vi "副屏设置.vi"() -> ()   [LabVIEW 2016, in "副屏.lvlib"]
uses:
  <vilib>/Utility/config.llb/NI_LVConfig.lvlib
panel:
  in  "ORP":bool caption="氨氮禁用"
  in  "启用副屏":bool=TRUE caption="氨氮禁用"
  in  "关闭":bool
  in  "底部状态栏显示信息":string="一体化微型水质监测系统"
  in  "流速":bool caption="氨氮禁用"
  in  "瞬时流量":bool caption="氨氮禁用"
  in  "湿度":bool=TRUE caption="氨氮禁用"
  in  "水位":bool caption="氨氮禁用"
  in  "室温":bool=TRUE caption="氨氮禁用"
  in  "CODCr":bool caption="氨氮禁用"
  in  "CODMn":bool caption="氨氮禁用"
  in  "总氮":bool caption="氨氮禁用"
  in  "总磷":bool caption="氨氮禁用"
  in  "氨氮":bool caption="氨氮禁用"
  in  "Turb":bool caption="氨氮禁用"
  in  "Cond":bool caption="氨氮禁用"
  in  "DO":bool caption="氨氮禁用"
  in  "pH":bool caption="氨氮禁用"
  in  "水温":bool caption="氨氮禁用"
  # "副屏显示信息设置"
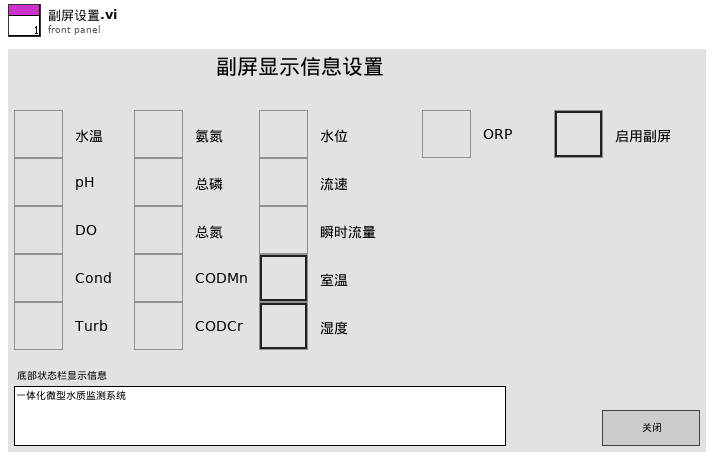
[diagram p1: front panel]
types:
  T1 = typedef "NI_LVConfig.lvlib/Config Data RefNum.ctl" = refnum<k1>
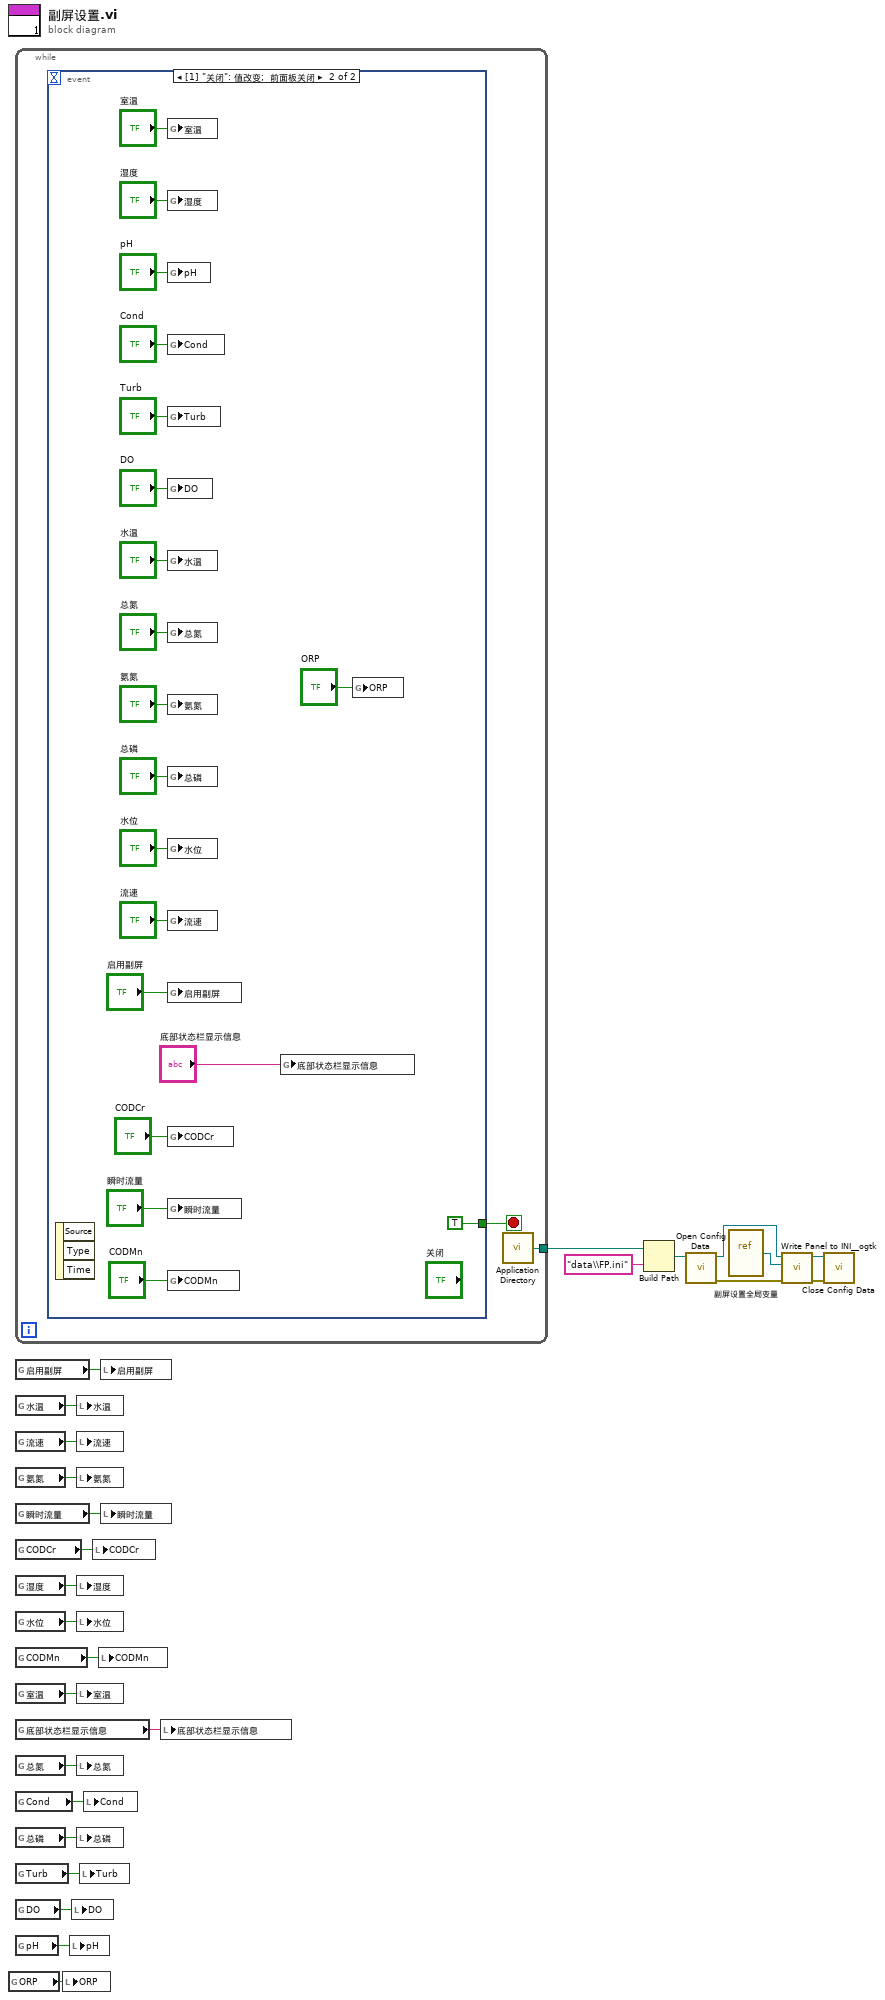
[diagram p0: block diagram]
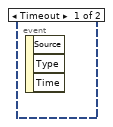
[diagram p2: hidden frame]
diagram:
  n1 = global read "副屏设置全局变量.vi" "ORP"() -> (w1:bool)
  n2 = while {
    tunnel: [w27] -> w3
    stop <- w28 stop-if-true
    n3 = event shown="[1] \"关闭\": 值改变;  前面板关闭" {
      selector: _ -> [_ _]
      dyn-events: _ -> [_ _]
      timeout: _ -> [_ _]
      tunnel: [_ TRUE] -> w28
      event Timeout {
        n4 = event-data() -> ()  [unwired: 1 in, 3 out]
      }
      event "关闭": Value Change; Panel Close {
        n5 = event-data() -> ()  [unwired: 1 in, 3 out]
        n6 = global write "副屏设置全局变量.vi" "室温"("室温") -> ()
        n7 = global write "副屏设置全局变量.vi" "湿度"("湿度") -> ()
        n8 = global write "副屏设置全局变量.vi" "pH"("pH") -> ()
        n9 = global write "副屏设置全局变量.vi" "Cond"("Cond") -> ()
        n10 = global write "副屏设置全局变量.vi" "Turb"("Turb") -> ()
        n11 = global write "副屏设置全局变量.vi" "DO"("DO") -> ()
        n12 = global write "副屏设置全局变量.vi" "水温"("水温") -> ()
        n13 = global write "副屏设置全局变量.vi" "总氮"("总氮") -> ()
        n14 = global write "副屏设置全局变量.vi" "氨氮"("氨氮") -> ()
        n15 = global write "副屏设置全局变量.vi" "总磷"("总磷") -> ()
        n16 = global write "副屏设置全局变量.vi" "水位"("水位") -> ()
        n17 = global write "副屏设置全局变量.vi" "流速"("流速") -> ()
        n18 = global write "副屏设置全局变量.vi" "启用副屏"("启用副屏") -> ()
        n19 = global write "副屏设置全局变量.vi" "CODCr"("CODCr") -> ()
        n20 = global write "副屏设置全局变量.vi" "瞬时流量"("瞬时流量") -> ()
        n21 = global write "副屏设置全局变量.vi" "CODMn"("CODMn") -> ()
        n22 = global write "副屏设置全局变量.vi" "底部状态栏显示信息"("底部状态栏显示信息") -> ()
        n23 = global write "副屏设置全局变量.vi" "ORP"("ORP") -> ()
      }
    }
    n24 = call <vilib>:"Application Directory.vi"() -> ("Application Directory"=w27:path)
  }
  n25 = global read "副屏设置全局变量.vi" "启用副屏"() -> (w2:bool)
  n26 = global read "副屏设置全局变量.vi" "水温"() -> (w26:bool)
  n27 = global read "副屏设置全局变量.vi" "流速"() -> (w20:bool)
  n28 = global read "副屏设置全局变量.vi" "氨氮"() -> (w25:bool)
  n29 = global read "副屏设置全局变量.vi" "瞬时流量"() -> (w18:bool)
  n30 = global read "副屏设置全局变量.vi" "CODCr"() -> (w24:bool)
  n31 = global read "副屏设置全局变量.vi" "湿度"() -> (w17:bool)
  n32 = global read "副屏设置全局变量.vi" "水位"() -> (w23:bool)
  n33 = global read "副屏设置全局变量.vi" "CODMn"() -> (w22:bool)
  n34 = global read "副屏设置全局变量.vi" "室温"() -> (w14:bool)
  n35 = global read "副屏设置全局变量.vi" "底部状态栏显示信息"() -> (w21:string)
  n36 = global read "副屏设置全局变量.vi" "总氮"() -> (w15:bool)
  n37 = global read "副屏设置全局变量.vi" "Cond"() -> (w19:bool)
  n38 = global read "副屏设置全局变量.vi" "总磷"() -> (w12:bool)
  n39 = global read "副屏设置全局变量.vi" "Turb"() -> (w13:bool)
  n40 = global read "副屏设置全局变量.vi" "DO"() -> (w16:bool)
  n41 = global read "副屏设置全局变量.vi" "pH"() -> (w11:bool)
  n42 = local write "ORP"(w1) -> ()
  n43 = local write "pH"(w11) -> ()
  n44 = local write "DO"(w16) -> ()
  n45 = local write "水温"(w26) -> ()
  n46 = local write "流速"(w20) -> ()
  n47 = local write "氨氮"(w25) -> ()
  n48 = local write "湿度"(w17) -> ()
  n49 = local write "水位"(w23) -> ()
  n50 = local write "室温"(w14) -> ()
  n51 = local write "总氮"(w15) -> ()
  n52 = local write "总磷"(w12) -> ()
  n53 = local write "Turb"(w13) -> ()
  n54 = local write "Cond"(w19) -> ()
  n55 = local write "CODCr"(w24) -> ()
  n56 = local write "CODMn"(w22) -> ()
  n57 = local write "启用副屏"(w2) -> ()
  n58 = local write "瞬时流量"(w18) -> ()
  n59 = local write "底部状态栏显示信息"(w21) -> ()
  n60 = Build Path(base path=w3, name or relative path="data\\FP.ini" ("名称或相对路径")) -> (appended path=w5:path)
  n61 = call <vilib>:"Open Config Data.vi"("configuration file path"=w5) -> ("error out"=w9:errorcluster, "refnum"=w6:T1)  [unwired: 8 in, 1 out]
  n62 = vi-ref "副屏设置全局变量.vi"() -> (w7:refnum<vi>)
  n63 = call <userlib>:"Write Panel to INI__ogtk.vi"("error in (no error)"=w9, "VI ref"=w7, "refnum"=w6) -> ("error out"=w10:errorcluster, "refnum out"=w8:T1)  [unwired: 7 in]
  n64 = call <vilib>:"Close Config Data.vi"("error in (no error)"=w10, "refnum"=w8) -> ()  [unwired: 8 in, 2 out]
